vi "Analyze Packet by UART.vi"(0 "VISA resource name in":refnum<visa-resource-name>, 1 "error in":errorcluster caption="error out") -> (2 "VISA resource name out":refnum<visa-resource-name>, 3 "Packet":u8[](array[numeric]), 4 "error out":errorcluster)   [LabVIEW 2011]
panel:
  out "85?":bool
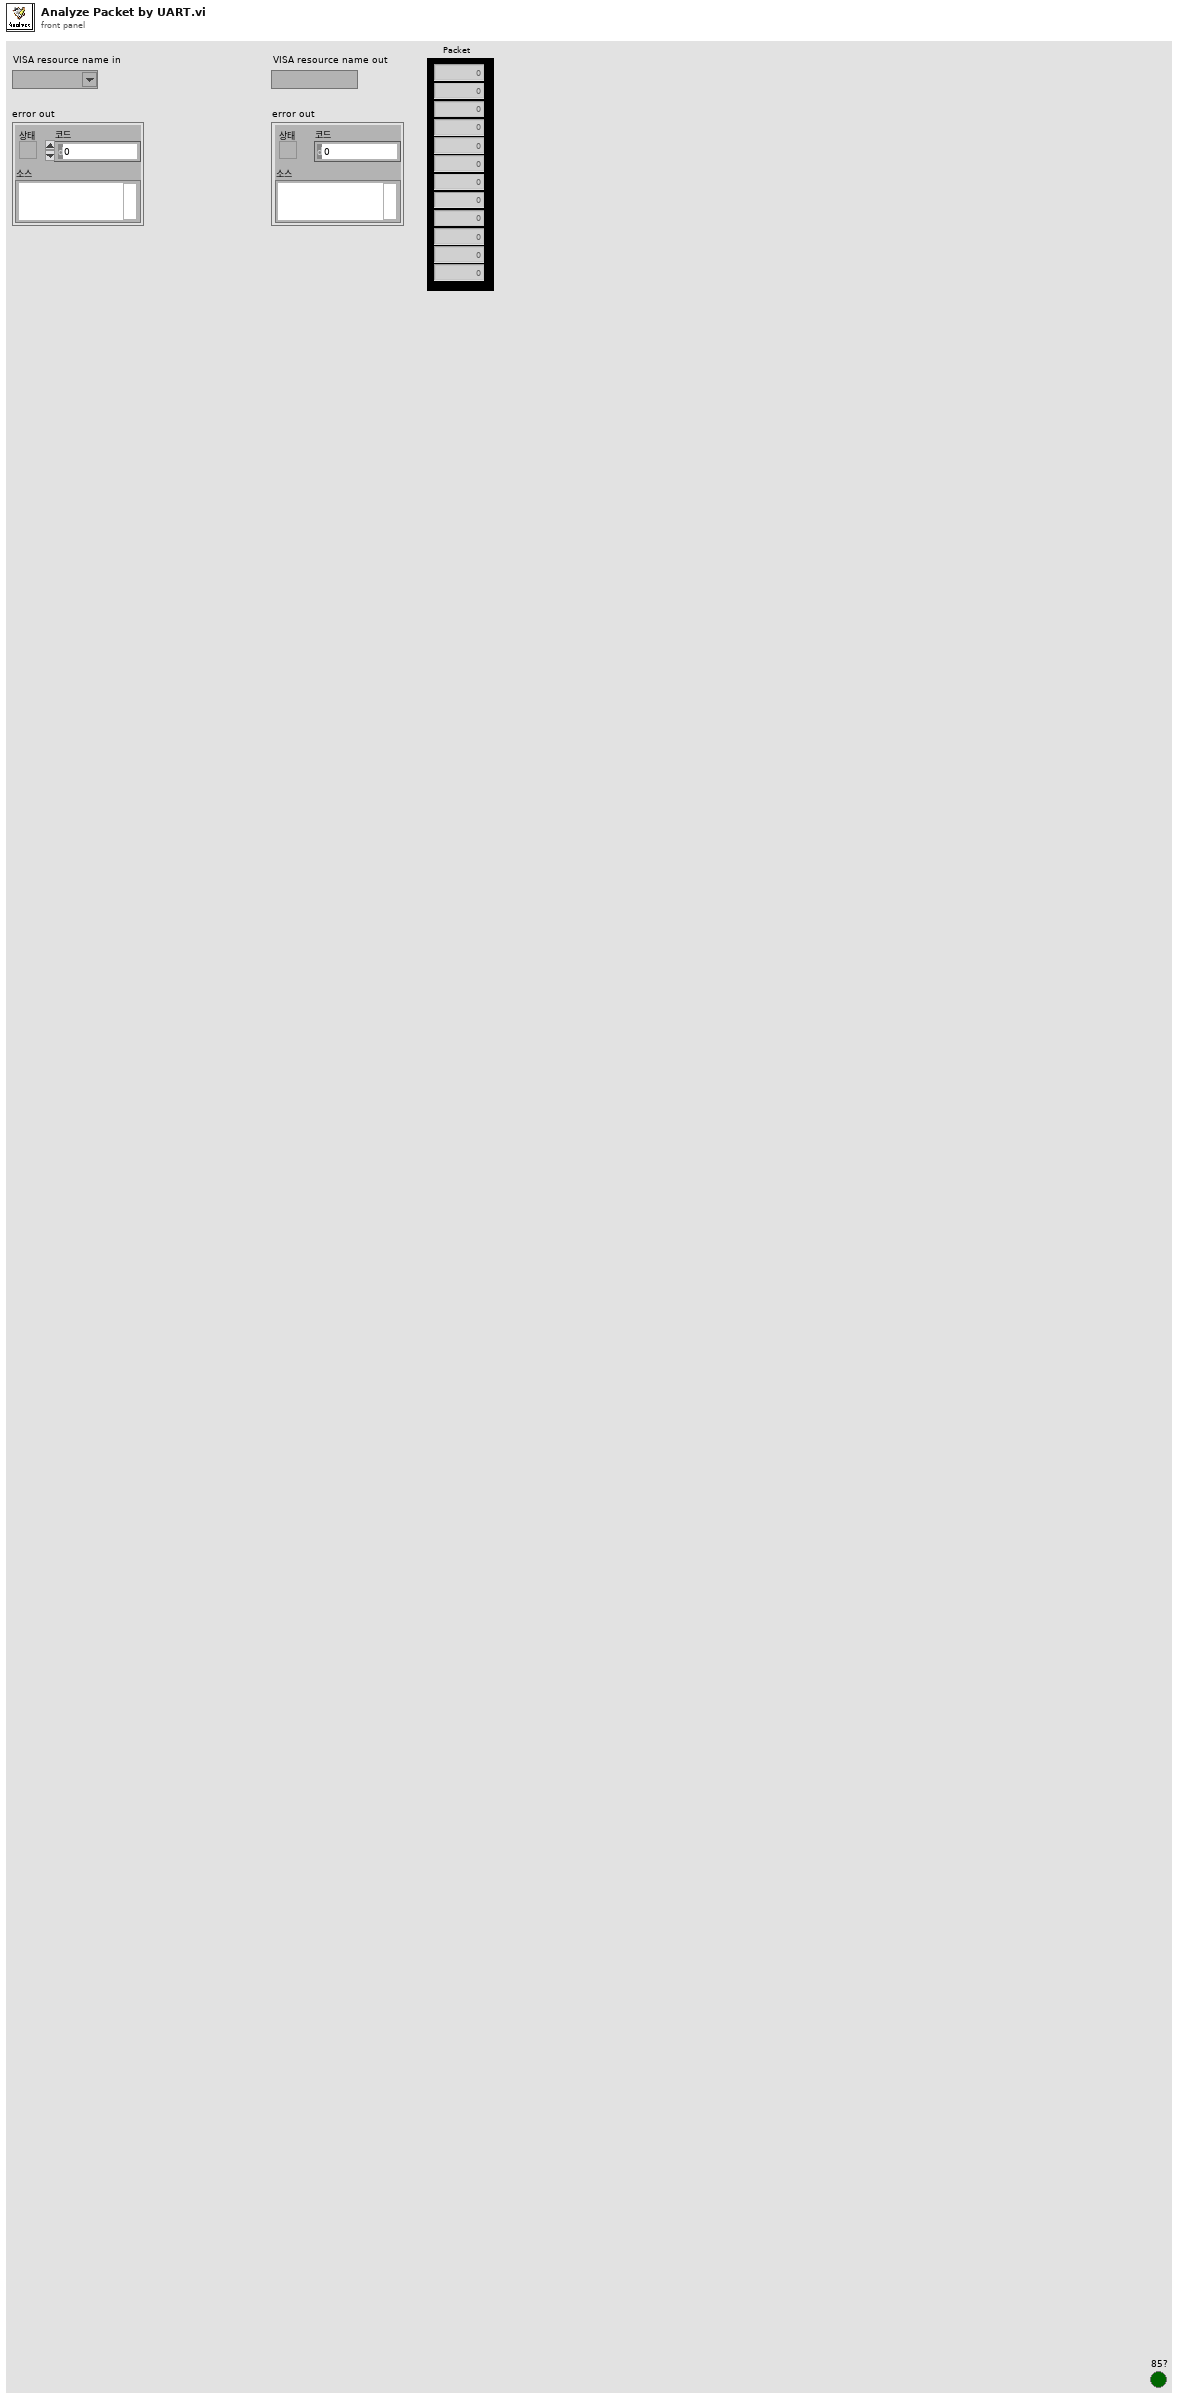
[diagram p1: front panel]
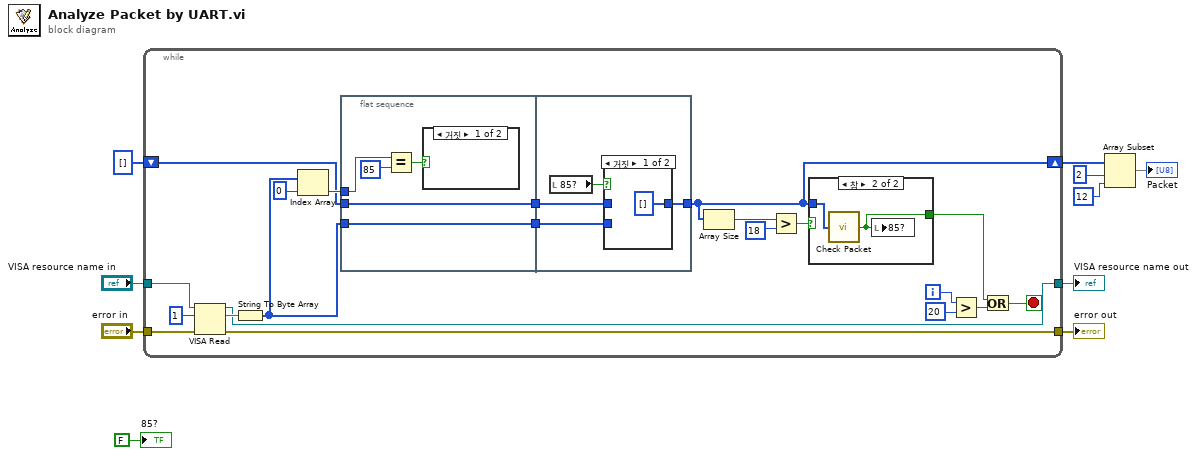
[diagram p0: block diagram]
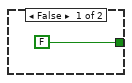
[diagram p2: hidden frame]
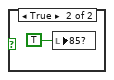
[diagram p3: hidden frame]
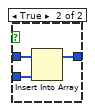
[diagram p4: hidden frame]
diagram:
  n1 = while {
    shift-right: [w12] -> w3
    shift-left: u8[] [] -> [w16]
    tunnel: "VISA resource name in" -> [w31]
    tunnel: [w22] -> w7
    tunnel: "error in" -> [w30]
    tunnel: [w23] -> w8
    i -> [w27]
    stop <- w24 stop-if-true
    n2 = VISA Read(VISA resource name=w31, byte count=u32 1 ("바이트 카운트"), error in (no error)=w30) -> (VISA resource name out=w22:refnum<visa-resource-name>, read buffer=w29:string, error out=w23:errorcluster)  [unwired: 1 out]
    n3 = String To Byte Array(string=w29) -> (unsigned byte array=w17:u8[])
    n4 = Index Array(array=w17, index=0 ("인덱스")) -> (element=w20:u8)
    n5 = flat-sequence {
      tunnel: w20 -> [w39]
      tunnel: w17 -> [w35]
      tunnel: w16 -> [w36]
      tunnel: [w36] -> w15
      tunnel: [w35] -> w14
      tunnel: w15 -> [w44]
      tunnel: w14 -> [w43]
      tunnel: [w41] -> w12
      frame #0 {
        n6 = Equal?(x=w39, y=u8 85) -> (x = y?=w37:bool)
        n7 = case shown="거짓" w37 {
          frame False {
          }
          frame True {
            n8 = local write "85?"(TRUE) -> ()
          }
        }
      }
      frame #1 {
        n9 = local read "85?"() -> (w42:bool)
        n10 = case shown="거짓" w42 {
          tunnel: w44 -> [_ w48]
          tunnel: w43 -> [_ w47]
          tunnel: [u8[] [] w46] -> w41
          frame False {
          }
          frame True {
            n11 = Insert Into Array(array=w48, new element=w47) -> (w46:u8[])  [unwired: 1 in]
          }
        }
      }
    }
    n12 = Array Size(array=w12) -> (size(s)=w28:i32)
    n13 = Greater?(x=w28, y=18) -> (0:w13:bool)
    n14 = case shown="참" w13 {
      tunnel: w12 -> [_ w34]
      tunnel: [FALSE ("Packet?") w33] -> w11
      frame False {
      }
      frame True {
        n15 = call "Check Packet.vi"("Serial"=w34) -> ("Packet?"=w33:bool)
        n16 = local write "85?"(w33) -> ()
      }
    }
    n17 = Greater?(x=w27, y=20) -> (0:w25:bool)
    n18 = Or(x=w11, y=w25) -> (x .or. y?=w24:bool)
  }
  "error out" <- w8
  "VISA resource name out" <- w7
  n19 = Array Subset(array=w3, index=2 ("인덱스"), length=12 ("인덱스")) -> (→"Packet":u8[])
  "85?" <- FALSE ("85?")
